vi "Read State.vi"(8 "error in (no error)":errorcluster, 11 "Context in":refnum<class "Context.lvclass">) -> (0 "error out":errorcluster, 2 "State":refnum<class "State Pattern.lvclass">, 3 "Context out":refnum<class "Context.lvclass">)   [LabVIEW 2021, in "Context.lvclass"]
uses:
  Context.lvclass
  State Pattern/State Pattern.lvclass
  Context.lvclass/Context.ctl
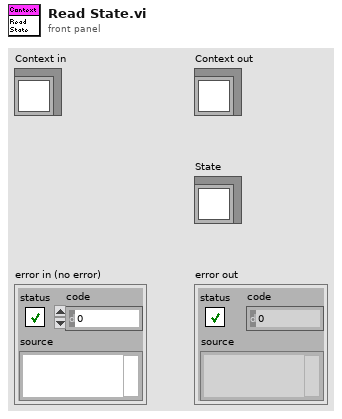
[diagram p1: front panel]
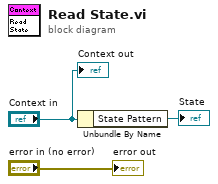
[diagram p0: block diagram]
diagram:
  n1 = Unbundle By Name("Context in") -> ("State Pattern"=→"State":refnum<class "State Pattern.lvclass">)
  "error out" <- "error in (no error)"
  "Context out" <- "Context in"
